vi "Tidy_Graph_v00.vi"(0 "パラメ B":T3={"Offset Error"=-0.0051412429378531075, "Gain Error"=1, "P Gain"=1, "P Bit Shift"=1, "I Bit Shift"=17, "I2 Bit Shift"=-11, "I Gain"=-10, "I2 Gain"=-27, "Lock Threshold"=13, "Lock"=FALSE, "Hold"=FALSE, "Scan Frequency"=8, "Scan Bit Shift"=-5, "Gains -ve "=TRUE, "Pre- Offset Error"=-5.0} {"Pre- Offset Error" scale=-0.01..0.01 scale format="%#_5f"; "Scan Frequency" scale=1.0..30.0; "I2 Gain" scale=0.0..10.0; "I Gain" scale=0.0..50.0; "P Gain" scale=0.0..50.0; "Offset Error" scale=-0.01..0.01 scale format="%#_5f"}, 1 "パラメ A":T3={"Offset Error"=-0.0051412429378531075, "Gain Error"=1, "P Gain"=1, "P Bit Shift"=1, "I Bit Shift"=17, "I2 Bit Shift"=-11, "I Gain"=-10, "I2 Gain"=-27, "Lock Threshold"=13, "Lock"=FALSE, "Hold"=FALSE, "Scan Frequency"=8, "Scan Bit Shift"=-5, "Gains -ve "=TRUE, "Pre- Offset Error"=-5.0} {"Pre- Offset Error" scale=-0.01..0.01 scale format="%#_5f"; "Scan Frequency" scale=1.0..30.0; "I2 Gain" scale=0.0..10.0; "I Gain" scale=0.0..50.0; "P Gain" scale=0.0..50.0; "Offset Error" scale=-0.01..0.01 scale format="%#_5f"}, 3 "Safety First Graph":T1, 5 "EPR BS":T3={"Offset Error"=-0.0051412429378531075, "Gain Error"=1, "P Gain"=1, "P Bit Shift"=1, "I Bit Shift"=17, "I2 Bit Shift"=-11, "I Gain"=-10, "I2 Gain"=-27, "Lock Threshold"=13, "Lock"=FALSE, "Hold"=FALSE, "Scan Frequency"=8, "Scan Bit Shift"=-5, "Gains -ve "=TRUE, "Pre- Offset Error"=-5.0} {"Pre- Offset Error" scale=-0.01..0.01 scale format="%#_5f"; "Scan Frequency" scale=1.0..30.0; "I2 Gain" scale=0.0..10.0; "I Gain" scale=0.0..50.0; "P Gain" scale=0.0..50.0; "Offset Error" scale=-0.01..0.01 scale format="%#_5f"}, 7 "Graph BS":T3={"Offset Error"=-0.0051412429378531075, "Gain Error"=1, "P Gain"=1, "P Bit Shift"=1, "I Bit Shift"=17, "I2 Bit Shift"=-11, "I Gain"=-10, "I2 Gain"=-27, "Lock Threshold"=13, "Lock"=FALSE, "Hold"=FALSE, "Scan Frequency"=8, "Scan Bit Shift"=-5, "Gains -ve "=TRUE, "Pre- Offset Error"=-5.0} {"Pre- Offset Error" scale=-0.01..0.01 scale format="%#_5f"; "Scan Frequency" scale=1.0..30.0; "I2 Gain" scale=0.0..10.0; "I Gain" scale=0.0..50.0; "P Gain" scale=0.0..50.0; "Offset Error" scale=-0.01..0.01 scale format="%#_5f"}, 9 "Homodyne A":T12={"Pre-Offset p Error"=-0.0051412429378531075, "Gain Error x"=1, "P Gain"=1, "P Bit Shift"=1, "I Bit Shift"=17, "I2 Bit Shift"=-11, "I Gain"=-10, "I2 Gain"=-27, "Lock Threshold"=13, "Lock"=FALSE, "Hold"=FALSE, "Scan Frequency"=8, "Scan Bit Shift"=-5, "Gains -ve "=TRUE, "Pre- Offset x"=-5.0, "Lock Angle (θ)"=0.0, "Gain Error p\n\n"=1} {"Lock Angle (θ)" min=-90.0 max=90.0 scale=-90.0..90.0 scale format="%#_2g"; "Pre- Offset x" scale=-0.01..0.01 scale format="%#_5f"; "Scan Frequency" scale=1.0..30.0; "I2 Gain" scale=0.0..10.0; "I Gain" scale=0.0..50.0; "P Gain" scale=0.0..50.0; "Pre-Offset p Error" scale=-0.01..0.01 scale format="%#_5f"}, 11 "Homodyne B":T12={"Pre-Offset p Error"=-0.0051412429378531075, "Gain Error x"=1, "P Gain"=1, "P Bit Shift"=1, "I Bit Shift"=17, "I2 Bit Shift"=-11, "I Gain"=-10, "I2 Gain"=-27, "Lock Threshold"=13, "Lock"=FALSE, "Hold"=FALSE, "Scan Frequency"=8, "Scan Bit Shift"=-5, "Gains -ve "=TRUE, "Pre- Offset x"=-5.0, "Lock Angle (θ)"=0.0, "Gain Error p\n\n"=1} {"Lock Angle (θ)" min=-90.0 max=90.0 scale=-90.0..90.0 scale format="%#_2g"; "Pre- Offset x" scale=-0.01..0.01 scale format="%#_5f"; "Scan Frequency" scale=1.0..30.0; "I2 Gain" scale=0.0..10.0; "I Gain" scale=0.0..50.0; "P Gain" scale=0.0..50.0; "Pre-Offset p Error" scale=-0.01..0.01 scale format="%#_5f"}, 12 "Graph Extras":T22={"Error Bit Sh."={"パラメ A"=0, "パラメ B"=0, "EPR BS"=0, "Graph BS"=0, "HD A x"=0, "HD A p"=0, "HD B x"=0, "HD B p"=0}, "I Max value"=20000, "I2 Max value"=20000, "Scan Offset"={"パラメ A"=0.0, "パラメ B"=0.0, "EPR BS"=0.0, "Graph BS"=0.0, "HD A"=0.0, "HD B"=0.0}, "Scan Ampl."={"パラメ A"=0.0, "パラメ B"=0.0, "EPR BS"=0.0, "Graph BS"=0.0, "HD A"=0.0, "HD B"=0.0}, "Scan-PII thresh"={"パラメ A"=1000, "パラメ B"=1000, "EPR BS"=1000, "Graph BS"=1000, "Homodyne A"=0, "Homodyne B"=0}, "Re-Scan thresh"={"パラメ A"=0, "パラメ B"=0, "EPR BS"=0, "Graph BS"=0, "Homodyne A"=0, "Homodyne B"=0}, "Post-Offset"={"HD A x"=0.0, "HD A p"=0.0, "HD B x"=0.0, "HD B p"=0.0}}, 13 "Scope+Safety":T21={"Safety First"={"lim reset"=FALSE, "no limit"=FALSE, "pos slew rate * dt"=100, "neg slew rate * dt"=-100, "Count(Ticks)"=0}, "Scope IPs"={"Trigger Direction"=enum."minus-plus", "Trigger Delay (ms)"=0.0, "Aquisition Rate (kHz)"=4000.0, "Trigger Offset (V)"=0.0, "Scale Offset"={"Scaling"={"Error signal"=1, "Output"=1, "DC Monitor"=1, "Threshold"=1}, "Offset"={"Error Signal"=0, "Output"=0, "DC Monitor"=0, "Threshold"=0}}}}, 14 "Hold All":T20) -> (15 "Control Graph to FPGA":T19={"PII In 1"={"Lock"=FALSE, "Hold"=FALSE, "P Gain"=0, "P BS"=-5, "I Gain"=0, "I BS"=-10, "I2 G"=0, "I2 BS"=-26, "Scan Amp"=0, "Scan Off"=0, "Scan FS"=0, "SFS BS"=0, "I Max value"=10000, "I2 Max value"=10000, "Scope.Offset"=0, "Trigger Direction"=enum."either", "Scan-PII thresh"=0}, "PII In 2"={"Lock"=FALSE, "Hold"=FALSE, "P Gain"=0, "P BS"=-10, "I Gain"=0, "I BS"=-10, "I2 G"=0, "I2 BS"=-26, "Scan Amp"=0, "Scan Off"=0, "Scan FS"=0, "SFS BS"=0, "I Max value"=10000, "I2 Max value"=10000, "Scope.Offset"=0, "Trigger Direction"=enum."either", "Scan-PII thresh"=0}, "PII In 3"={"Lock"=FALSE, "Hold"=FALSE, "P Gain"=0, "P BS"=-10, "I Gain"=0, "I BS"=-10, "I2 G"=0, "I2 BS"=-26, "Scan Amp"=0, "Scan Off"=0, "Scan FS"=0, "SFS BS"=0, "I Max value"=10000, "I2 Max value"=10000, "Scope.Offset"=0, "Trigger Direction"=enum."either", "Scan-PII thresh"=0}, "PII In 4"={"Lock"=FALSE, "Hold"=FALSE, "P Gain"=0, "P BS"=-10, "I Gain"=0, "I BS"=-10, "I2 G"=0, "I2 BS"=-26, "Scan Amp"=0, "Scan Off"=0, "Scan FS"=0, "SFS BS"=0, "I Max value"=10000, "I2 Max value"=10000, "Scope.Offset"=0, "Trigger Direction"=enum."either", "Scan-PII thresh"=0}, "PII In 5"={"Lock"=FALSE, "Hold"=FALSE, "P Gain"=0, "P BS"=-10, "I Gain"=0, "I BS"=-10, "I2 G"=0, "I2 BS"=-26, "Scan Amp"=0, "Scan Off"=0, "Scan FS"=0, "SFS BS"=0, "I Max value"=10000, "I2 Max value"=10000, "Scope.Offset"=0, "Trigger Direction"=enum."either", "Scan-PII thresh"=0}, "PII In 6"={"Lock"=FALSE, "Hold"=FALSE, "P Gain"=0, "P BS"=-10, "I Gain"=0, "I BS"=-10, "I2 G"=0, "I2 BS"=-26, "Scan Amp"=0, "Scan Off"=0, "Scan FS"=0, "SFS BS"=0, "I Max value"=10000, "I2 Max value"=10000, "Scope.Offset"=0, "Trigger Direction"=enum."either", "Scan-PII thresh"=0}, "Error scale"={"Pre-Offset"={"Pre-Offset 1"=2, "Pre-Offset 2"=0, "Pre-Offset 3"=0, "Pre-Offset 4"=0, "Pre-Offset 5"=2}, "Post-Offset "={"Offset 1"=0, "Offset 2"=300, "Offset 3"=0, "Offset 4"=0, "Offset 5"=0}, "Gains"={"Gain 1"=0, "Gain 2"=300, "Gain 3"=0, "Gain 4"=0, "Gain 5"=0}, "Bit Shifts"={"Bit Shift 1"=0, "Bit Shift 2"=300, "Bit Shift 3"=0, "Bit Shift 4"=0, "Bit Shift 5"=0}}, "Lock Thresh"={"EPR"=2, "HD A"=0, "HD B"=40}, "Re-Scan Thresh"={"EPR"=2, "HD A"=0, "HD B"=40}, "Theta"={"HD A Sin Theta"=0, "HD A Cos Theta"=0, "HD B Sin Theta"=0, "HD B Cos Theta"=0}, "Safety First"={"lim reset"=FALSE, "no limit"=FALSE, "pos slew rate * dt"=10, "neg slew rate * dt"=-10, "Hold All"=FALSE, "Count(Ticks)"=0}})   [LabVIEW 2011]
doc: "The data structures from the User Interface need are rebundled here to match that of the FPGA_Cavity VI."
uses:
  Strict Type Defs/Slider and display.ctl
  Strict Type Defs/I16 white control.ctl
  Strict Type Defs/PII Gains.ctl
  Strict Type Defs/Lock or Hold.ctl
  Strict Type Defs/Safety First.ctl
  Strict Type Defs/Thresh slider.ctl
  Strict Type Defs/Scope and Safety.ctl
  Strict Type Defs/Hold All.ctl
  Strict Type Defs/PII individual.ctl
  Strict Type Defs/Error Scale 1SDI.ctl
  Strict Type Defs/Lock Thresh 1SDI.ctl
  Strict Type Defs/Theta graph.ctl
  Strict Type Defs/Lock Select.ctl
  Strict Type Defs/Control GUI Graph v00.ctl
  Strict Type Defs/I2 gain slider.ctl
  Strict Type Defs/Scan Freq Slider.ctl
  Strict Type Defs/Gains negative vertical.ctl
  Strict Type Defs/Graph Extras.ctl
  Strict Type Defs/Double Graph control.ctl
  Strict Type Defs/I16 Graph Control.ctl
  Strict Type Defs/theta.ctl
  Strict Type Defs/GUI HD Graph.ctl
panel:
  in  "Lock Select":T2=enum."Doubler"
  in  "Control Graph":T19={"PII In 1"={"Lock"=FALSE, "Hold"=FALSE, "P Gain"=0, "P BS"=-5, "I Gain"=0, "I BS"=-10, "I2 G"=0, "I2 BS"=-26, "Scan Amp"=0, "Scan Off"=0, "Scan FS"=0, "SFS BS"=0, "I Max value"=10000, "I2 Max value"=10000, "Scope.Offset"=0, "Trigger Direction"=enum."either", "Scan-PII thresh"=0}, "PII In 2"={"Lock"=FALSE, "Hold"=FALSE, "P Gain"=0, "P BS"=-10, "I Gain"=0, "I BS"=-10, "I2 G"=0, "I2 BS"=-26, "Scan Amp"=0, "Scan Off"=0, "Scan FS"=0, "SFS BS"=0, "I Max value"=10000, "I2 Max value"=10000, "Scope.Offset"=0, "Trigger Direction"=enum."either", "Scan-PII thresh"=0}, "PII In 3"={"Lock"=FALSE, "Hold"=FALSE, "P Gain"=0, "P BS"=-10, "I Gain"=0, "I BS"=-10, "I2 G"=0, "I2 BS"=-26, "Scan Amp"=0, "Scan Off"=0, "Scan FS"=0, "SFS BS"=0, "I Max value"=10000, "I2 Max value"=10000, "Scope.Offset"=0, "Trigger Direction"=enum."either", "Scan-PII thresh"=0}, "PII In 4"={"Lock"=FALSE, "Hold"=FALSE, "P Gain"=0, "P BS"=-10, "I Gain"=0, "I BS"=-10, "I2 G"=0, "I2 BS"=-26, "Scan Amp"=0, "Scan Off"=0, "Scan FS"=0, "SFS BS"=0, "I Max value"=10000, "I2 Max value"=10000, "Scope.Offset"=0, "Trigger Direction"=enum."either", "Scan-PII thresh"=0}, "PII In 5"={"Lock"=FALSE, "Hold"=FALSE, "P Gain"=0, "P BS"=-10, "I Gain"=0, "I BS"=-10, "I2 G"=0, "I2 BS"=-26, "Scan Amp"=0, "Scan Off"=0, "Scan FS"=0, "SFS BS"=0, "I Max value"=10000, "I2 Max value"=10000, "Scope.Offset"=0, "Trigger Direction"=enum."either", "Scan-PII thresh"=0}, "PII In 6"={"Lock"=FALSE, "Hold"=FALSE, "P Gain"=0, "P BS"=-10, "I Gain"=0, "I BS"=-10, "I2 G"=0, "I2 BS"=-26, "Scan Amp"=0, "Scan Off"=0, "Scan FS"=0, "SFS BS"=0, "I Max value"=10000, "I2 Max value"=10000, "Scope.Offset"=0, "Trigger Direction"=enum."either", "Scan-PII thresh"=0}, "Error scale"={"Pre-Offset"={"Pre-Offset 1"=2, "Pre-Offset 2"=0, "Pre-Offset 3"=0, "Pre-Offset 4"=0, "Pre-Offset 5"=2}, "Post-Offset "={"Offset 1"=0, "Offset 2"=300, "Offset 3"=0, "Offset 4"=0, "Offset 5"=0}, "Gains"={"Gain 1"=0, "Gain 2"=300, "Gain 3"=0, "Gain 4"=0, "Gain 5"=0}, "Bit Shifts"={"Bit Shift 1"=0, "Bit Shift 2"=300, "Bit Shift 3"=0, "Bit Shift 4"=0, "Bit Shift 5"=0}}, "Lock Thresh"={"EPR"=2, "HD A"=0, "HD B"=40}, "Re-Scan Thresh"={"EPR"=2, "HD A"=0, "HD B"=40}, "Theta"={"HD A Sin Theta"=0, "HD A Cos Theta"=0, "HD B Sin Theta"=0, "HD B Cos Theta"=0}, "Safety First"={"lim reset"=FALSE, "no limit"=FALSE, "pos slew rate * dt"=10, "neg slew rate * dt"=-10, "Hold All"=FALSE, "Count(Ticks)"=0}}
  in  "Safety First":T18
  # "PII Gains"
  # "Lock"
  # "Error Signal"
  # "Scan"
  # "PII Gains"
  # "Lock"
  # "Error Signal"
  # "Scan"
  # "PII Gains"
  # "Lock"
  # "Error Signal"
  # "Scan"
  # "PII Gains"
  # "Lock"
  # "Error Signal"
  # "Scan"
  # "PII Gains"
  # "Lock"
  # "Error Signal"
  # "Scan"
  # "PII Gains"
  # "Lock"
  # "Error Signal"
  # "Scan"
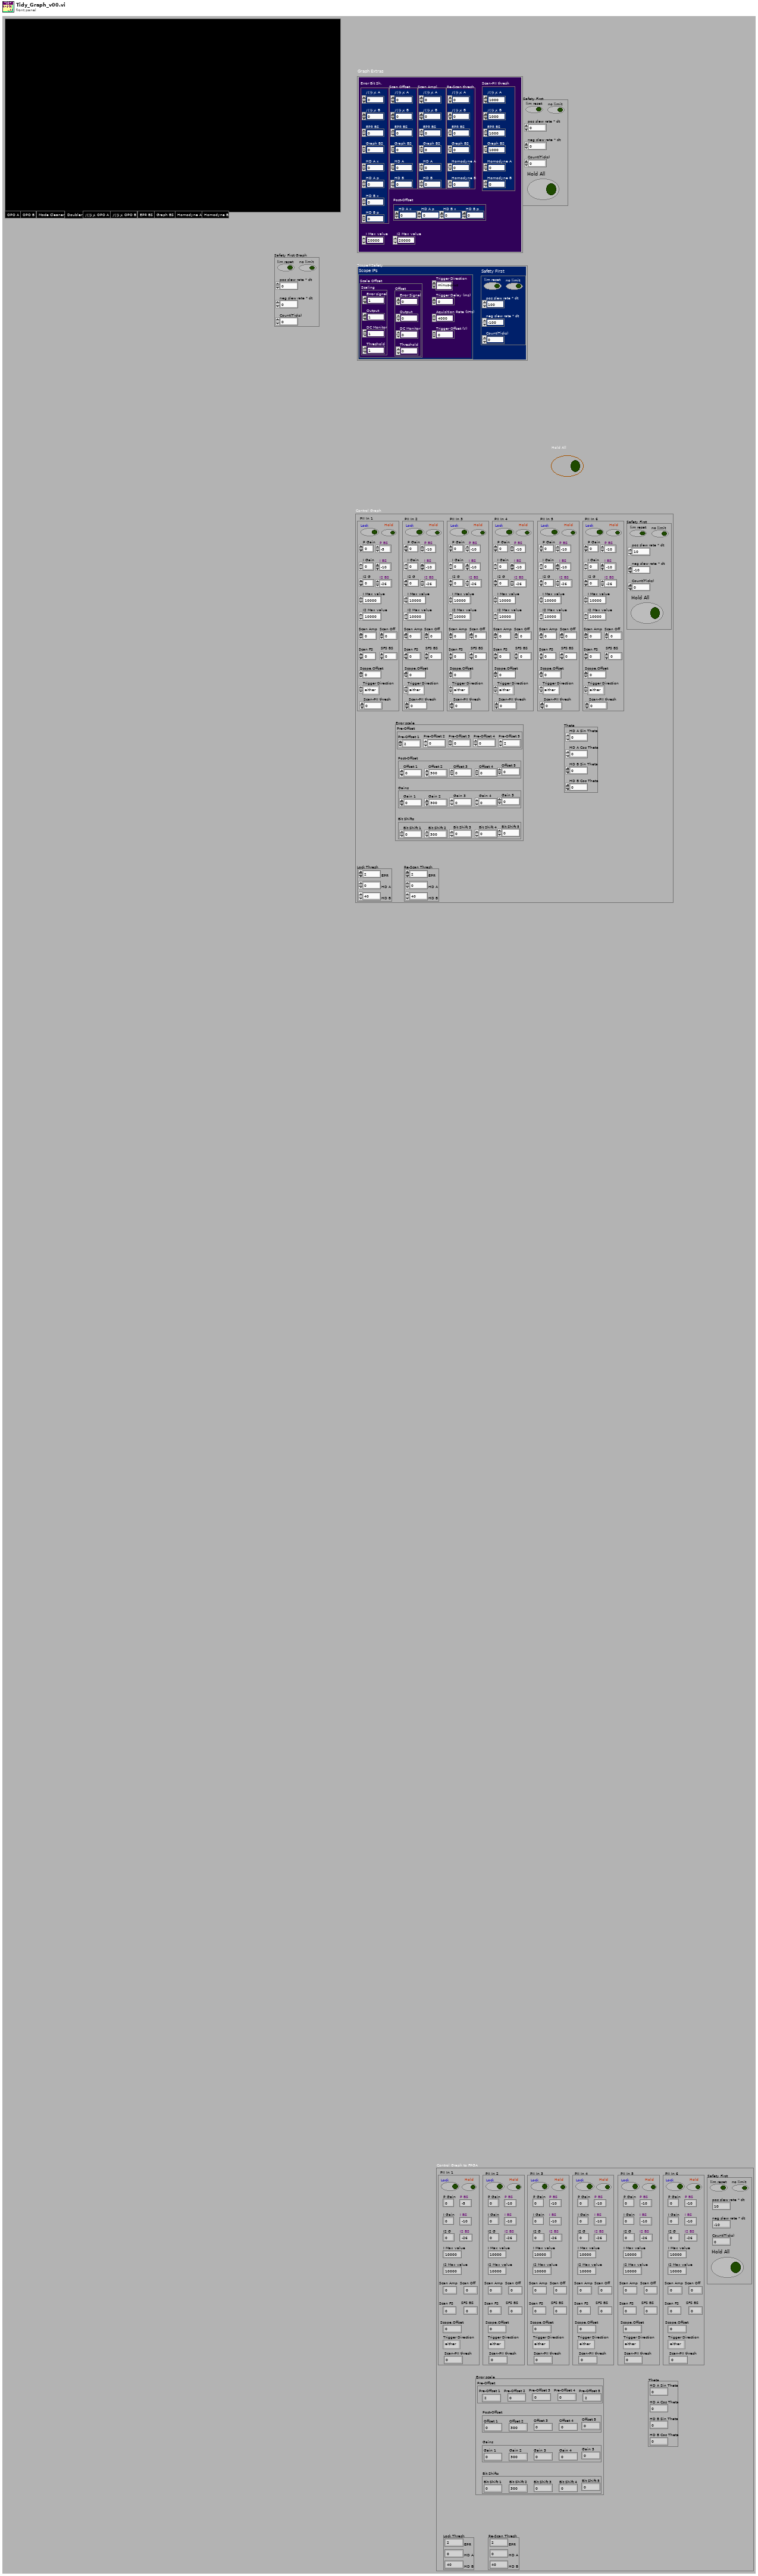
[diagram p1: front panel]
types:
  T1 = cluster{"lim reset":bool, "no limit":bool, "pos slew rate * dt":i16, "neg slew rate * dt":i16, "Count(Ticks)":u32}
  T2 = typedef "Lock Select.ctl" = enum32{"OPO A", "OPO B", "Mode Cleaner", "Doubler", "パラメ OPO A", "パラメ OPO B", "EPR BS", "Graph BS", "Homodyne A", "Homodyne B"}
  T3 = typedef "Control GUI Graph v00.ctl" = cluster{"Offset Error":T4, "Gain Error":T5, "P Gain":T6, "P Bit Shift":T5, "I Bit Shift":T5, "I2 Bit Shift":T5, "I Gain":T6, "I2 Gain":T7, "Lock Threshold":T8, "Lock":T9, "Hold":T9, "Scan Frequency":T10, "Scan Bit Shift":T5, "Gains -ve ":T11, "Pre- Offset Error":T4}
  T4 = typedef "Slider and display.ctl" = dbl
  T5 = typedef "I16 white control.ctl" = i16
  T6 = typedef "PII Gains.ctl" = i32
  T7 = typedef "I2 gain slider.ctl" = i32
  T8 = typedef "Thresh slider.ctl" = i16
  T9 = typedef "Lock or Hold.ctl" = bool
  T10 = typedef "Scan Freq Slider.ctl" = u16
  T11 = typedef "Gains negative vertical.ctl" = bool
  T12 = typedef "GUI HD Graph.ctl" = cluster{"Pre-Offset p Error":T4, "Gain Error x":T5, "P Gain":T6, "P Bit Shift":T5, "I Bit Shift":T5, "I2 Bit Shift":T5, "I Gain":T6, "I2 Gain":T7, "Lock Threshold":T8, "Lock":T9, "Hold":T9, "Scan Frequency":T10, "Scan Bit Shift":T5, "Gains -ve ":T11, "Pre- Offset x":T4, "Lock Angle (θ)":T13, "Gain Error p\n\n":T5}
  T13 = typedef "theta.ctl" = dbl
  T14 = typedef "PII individual.ctl" = cluster{"Lock":bool, "Hold":bool, "P Gain":i32, "P BS":i16, "I Gain":i32, "I BS":i16, "I2 G":i32, "I2 BS":i16, "Scan Amp":i16, "Scan Off":i16, "Scan FS":u16, "SFS BS":i16, "I Max value":i32, "I2 Max value":i32, "Scope.Offset":i16, "Trigger Direction":enum8{"either", "minus-plus", "plus-minus"}, "Scan-PII thresh":i16}
  T15 = typedef "Error Scale 1SDI.ctl" = cluster{"Pre-Offset":cluster{"Pre-Offset 1":i16, "Pre-Offset 2":i16, "Pre-Offset 3":i16, "Pre-Offset 4":i16, "Pre-Offset 5":i16}, "Post-Offset ":cluster{"Offset 1":i16, "Offset 2":i16, "Offset 3":i16, "Offset 4":i16, "Offset 5":i16}, "Gains":cluster{"Gain 1":i16, "Gain 2":i16, "Gain 3":i16, "Gain 4":i16, "Gain 5":i16}, "Bit Shifts":cluster{"Bit Shift 1":i16, "Bit Shift 2":i16, "Bit Shift 3":i16, "Bit Shift 4":i16, "Bit Shift 5":i16}}
  T16 = typedef "Lock Thresh 1SDI.ctl" = cluster{"EPR":i16, "HD A":i16, "HD B":i16}
  T17 = typedef "Theta graph.ctl" = cluster{"HD A Sin Theta":i32, "HD A Cos Theta":i32, "HD B Sin Theta":i32, "HD B Cos Theta":i32}
  T18 = typedef "Safety First.ctl" = cluster{"lim reset":bool, "no limit":bool, "pos slew rate * dt":i16, "neg slew rate * dt":i16, "Hold All":bool, "Count(Ticks)":u32}
  T19 = cluster{"PII In 1":T14, "PII In 2":T14, "PII In 3":T14, "PII In 4":T14, "PII In 5":T14, "PII In 6":T14, "Error scale":T15, "Lock Thresh":T16, "Re-Scan Thresh":T16, "Theta":T17, "Safety First":T18}
  T20 = typedef "Hold All.ctl" = bool
  T21 = typedef "Scope and Safety.ctl" = cluster{"Safety First":cluster{"lim reset":bool, "no limit":bool, "pos slew rate * dt":i16, "neg slew rate * dt":i16, "Count(Ticks)":u32}, "Scope IPs":cluster{"Trigger Direction":enum8{"either", "minus-plus", "plus-minus"}, "Trigger Delay (ms)":dbl, "Aquisition Rate (kHz)":dbl, "Trigger Offset (V)":dbl, "Scale Offset":cluster{"Scaling":cluster{"Error signal":i16, "Output":i16, "DC Monitor":i16, "Threshold":i16}, "Offset":cluster{"Error Signal":i16, "Output":i16, "DC Monitor":i16, "Threshold":i16}}}}
  T22 = typedef "Graph Extras.ctl" = cluster{"Error Bit Sh.":cluster{"パラメ A":i16, "パラメ B":i16, "EPR BS":i16, "Graph BS":i16, "HD A x":i16, "HD A p":i16, "HD B x":i16, "HD B p":i16}, "I Max value":i32, "I2 Max value":i32, "Scan Offset":T23, "Scan Ampl.":T23, "Scan-PII thresh":T24, "Re-Scan thresh":T24, "Post-Offset":cluster{"HD A x":dbl, "HD A p":dbl, "HD B x":dbl, "HD B p":dbl}}
  T23 = typedef "Double Graph control.ctl" = cluster{"パラメ A":dbl, "パラメ B":dbl, "EPR BS":dbl, "Graph BS":dbl, "HD A":dbl, "HD B":dbl}
  T24 = typedef "I16 Graph Control.ctl" = cluster{"パラメ A":i16, "パラメ B":i16, "EPR BS":i16, "Graph BS":i16, "Homodyne A":i16, "Homodyne B":i16}
  T25 = enum32{"OPO A", "OPO B", "Mode Cleaner", "Doubler", "パラメ OPO A", "パラメ OPO B", "EPR Beamsplitter", "Graph Beamsplitter", "Homodyne A", "Homodyne B"}
  T26 = typedef "Extras PII Graph HD.ctl" = cluster{"Error Bit Shift p":i16, "Scan Offset":dbl, "Scan Amplitude":dbl, "Scan-PII thresh":i16, "Re-Scan Thresh":i16, "I Max value":i32, "I2 Max value":i32, "Trigger Direction":enum8{"either", "minus-plus", "plus-minus"}, "Trigger Offset (V)":dbl, "Error Bit Shift x":i16, "Post-Offset p":dbl, "Post-Offset x":dbl}
  T27 = typedef "Extras PII Graph.ctl" = cluster{"Error Bit Shift":i16, "Scan Offset":dbl, "Scan Amplitude":dbl, "Scan-PII thresh":i16, "Re-Scan Thresh":i16, "I Max value":i32, "I2 Max value":i32, "Trigger Direction":enum8{"either", "minus-plus", "plus-minus"}, "Trigger Offset (V)":dbl}
  T28 = typedef "PII and Error Graph.ctl" = cluster{"Error individual":T29, "PII cavity":T14, "Lock Thresh":i16, "Re-Scan Thresh":i16}
  T29 = typedef "Errors Converted Graph.ctl" = cluster{"Error Pre Offset":i16, "Error Offset":i16, "Error Gain":i16, "Error Bit Shift":i16}
  T30 = typedef "PII and Error Graph HD.ctl" = cluster{"Error individual":T31, "PII cavity":T14, "Lock Thresh":i16, "Re-Scan Thresh":i16, "Sin Theta":i32, "Cos Theta":i32}
  T31 = typedef "Errors Converted Graph HD.ctl" = cluster{"Error Pre Offset x":i16, "Error Offset x":i16, "Error Gain x":i16, "Error Bit Shift x":i16, "Error Pre Offset p":i16, "Error Offset p":i16, "Error Gain p":i16, "Error Bit Shift p":i16}
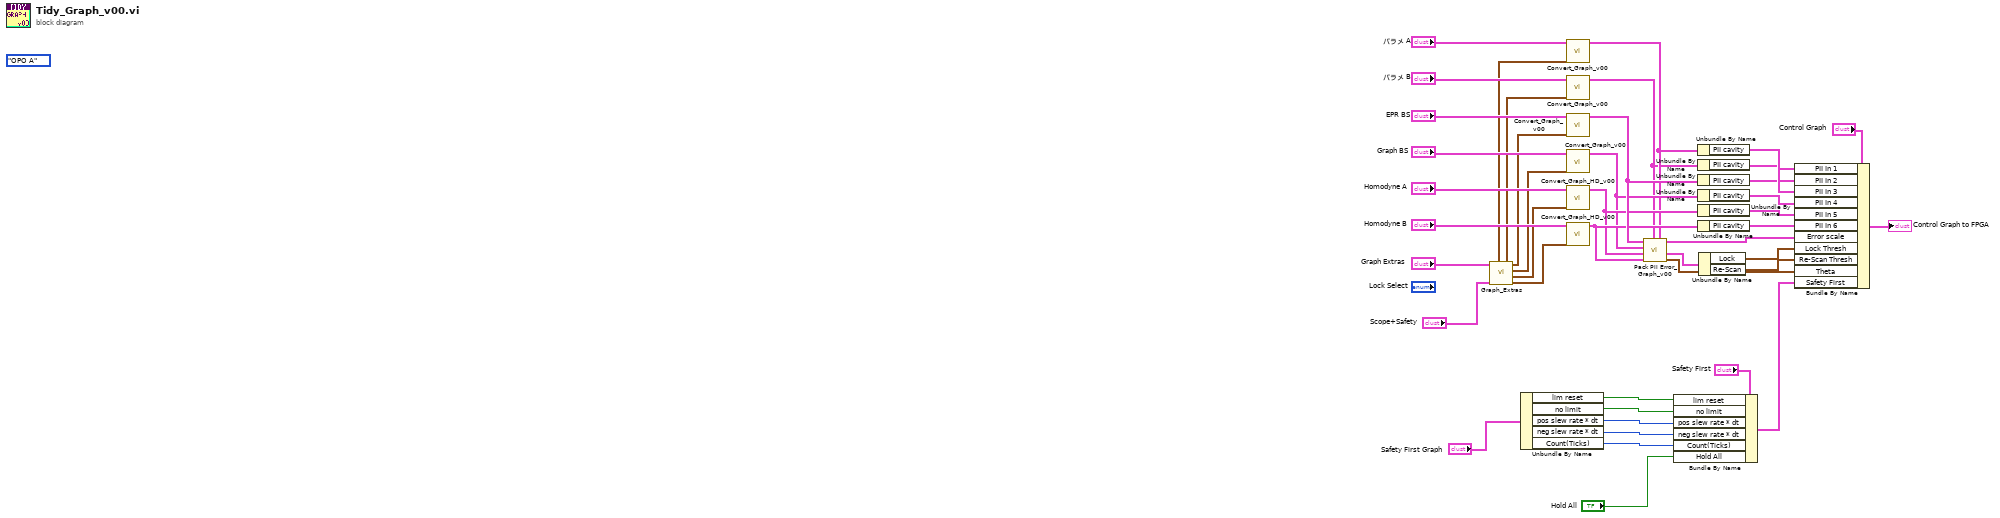
[diagram p0: block diagram]
diagram:
  (unwired) T25."OPO A" ("Tab Control")
  n1 = call "Graph_Extras.vi"("Scope+Safety"="Scope+Safety", "Graph Extras"="Graph Extras") -> ("Extras Homodyne B"=w17:T26, "Extras Homodyne A"=w18:T26, "Extras Graph"=w19:T27, "Extras EPR BS"=w20:T27, "Extras パラメ B"=w21:T27, "Extras パラメ A"=w22:T27)  [unwired: 4 in]
  n2 = Unbundle By Name("Safety First Graph") -> ("lim reset"=w37:bool, "no limit"=w36:bool, "pos slew rate * dt"=w35:i16, "neg slew rate * dt"=w34:i16, "Count(Ticks)"=w33:u32)
  n3 = call "Convert_Graph_v00.vi"("Extras PII"=w22, "PII Control"="パラメ A") -> ("PII+Error"=w16:T28)  [unwired: 9 in]
  n4 = call "Convert_Graph_v00.vi"("Extras PII"=w21, "PII Control"="パラメ B") -> ("PII+Error"=w15:T28)  [unwired: 9 in]
  n5 = call "Convert_Graph_v00.vi"("Extras PII"=w20, "PII Control"="EPR BS") -> ("PII+Error"=w42:T28)  [unwired: 9 in]
  n6 = call "Convert_Graph_v00.vi"("Extras PII"=w19, "PII Control"="Graph BS") -> ("PII+Error"=w39:T28)  [unwired: 9 in]
  n7 = call "Convert_Graph_HD_v00.vi"("Extras Homodyne"=w18, "PII Control"="Homodyne A") -> ("PII+Error"=w40:T30)  [unwired: 9 in]
  n8 = call "Convert_Graph_HD_v00.vi"("Extras Homodyne"=w17, "PII Control"="Homodyne B") -> ("PII+Error"=w41:T30)  [unwired: 9 in]
  n9 = call "Pack PII Error_Graph_v00.vi"("PII+Error pump A"=w16, "PII+Error pump B"=w15, "PII+Error HD B"=w41, "PII+Error HD A"=w40, "PII+Error Graph BS"=w39, "PII+Error EPR BS"=w42) -> ("Theta"=w10:T17, "Thresholds"=w11:cluster{"Lock":T16, "Re-Scan":T16}, "Error packed"=w12:T15)  [unwired: 3 in]
  n10 = Bundle By Name(cluster="Safety First", "lim reset"=w37, "no limit"=w36, "pos slew rate * dt"=w35, "neg slew rate * dt"=w34, "Count(Ticks)"=w33, "Hold All"="Hold All") -> (w29:T18)
  n11 = Unbundle By Name(w16) -> ("PII cavity"=w9:T14)
  n12 = Unbundle By Name(w15) -> ("PII cavity"=w8:T14)
  n13 = Unbundle By Name(w42) -> ("PII cavity"=w7:T14)
  n14 = Unbundle By Name(w39) -> ("PII cavity"=w6:T14)
  n15 = Unbundle By Name(w40) -> ("PII cavity"=w5:T14)
  n16 = Unbundle By Name(w41) -> ("PII cavity"=w4:T14)
  n17 = Unbundle By Name(w11) -> ("Lock"=w14:T16, "Re-Scan"=w13:T16)
  n18 = Bundle By Name(cluster="Control Graph", "PII In 1"=w9, "PII In 2"=w8, "PII In 3"=w7, "PII In 4"=w6, "PII In 5"=w5, "PII In 6"=w4, "Error scale"=w12, "Lock Thresh"=w14, "Re-Scan Thresh"=w13, "Theta"=w10, "Safety First"=w29) -> (→"Control Graph to FPGA":T19)
